vi "SET MARK MODE.vi"(8 "error in (no error)":errorcluster, 10 "mark mode":string, 11 "Domino Laser module Class in":refnum<class "Domino Laser module Class.lvclass">) -> (0 "error out":errorcluster, 3 "Domino Laser module Class out":refnum<class "Domino Laser module Class.lvclass">)   [LabVIEW 2015, in "Domino LM.lvlib" / "Domino Laser module Class.lvclass"]
uses:
  CTRLS/Domino Laser module Class.lvclass
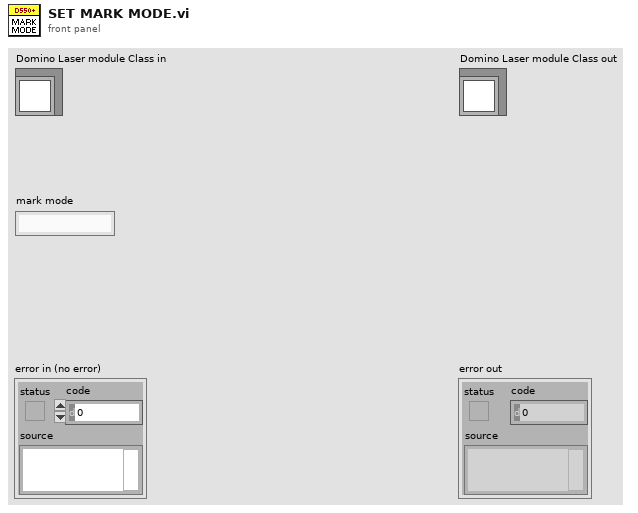
[diagram p1: front panel]
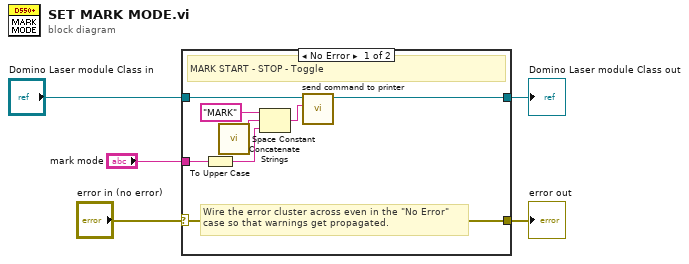
[diagram p0: block diagram]
diagram:
  n1 = case shown="No Error" "error in (no error)" {
    selector: "error in (no error)" -> [w13 w15]
    tunnel: [w13 w15] -> w4
    tunnel: [w6 w14] -> w2
    tunnel: "Domino Laser module Class in" -> [w7 w14]
    tunnel: "mark mode" -> [w12 _]
    frame No Error {
      # "Wire the error cluster across even in the \"No Error\"\ncase so that warnings get propagated."
      # "MARK START - STOP - Toggle"
      n2 = To Upper Case(1:w12) -> (0:w11:string)
      n3 = call <vilib>:"Space Constant.vi"() -> ("String"=w9:string)
      n4 = Concatenate Strings("MARK" ("string"), w9, w11) -> (w8:string)
      n5 = call "send command to printer.vi"("command to be sent"=w8, "Domino Laser module Class in"=w7) -> ("Domino Laser module Class out"=w6:refnum<class "Domino Laser module Class.lvclass">)  [unwired: 6 in, 3 out]
    }
    frame Error {
    }
  }
  "error out" <- w4
  "Domino Laser module Class out" <- w2
